vi "Re-Populate Tree.vi"(8 "error in":errorcluster, 9 "Tags map":refnum<vi>, 10 "Data in":string[][](array[string]), 11 "TreeControl in":refnum<vi>) -> (0 "error out":errorcluster)   [LabVIEW 2025, in "CAN-LIN Raw Bus Capture UI.lvlib"]
uses:
  CAN-LIN Raw Bus Capture UI.lvlib
  <vilib>/Utility/error.llb/whitespace.ctl
  <vilib>/Utility/error.llb/Trim Whitespace One-Sided.vi
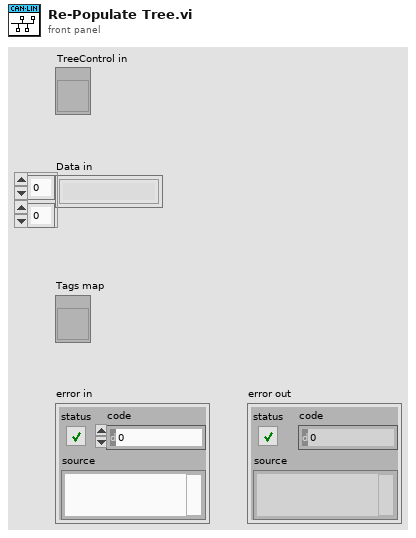
[diagram p1: front panel]
types:
  T1 = typedef "whitespace.ctl" = u16
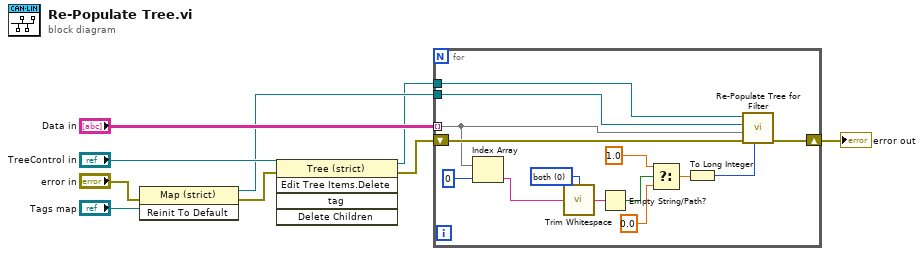
[diagram p0: block diagram]
diagram:
  n1 = invoke class="Map (strict)" method="Reinit To Default"(reference="Tags map", error in="error in") -> (reference out=w4:refnum<vi>, error out=w5:errorcluster)  [unwired: 1 in, 1 out]
  n2 = invoke class="Tree (strict)" method="Edit Tree Items.Delete"(reference="TreeControl in", error in=w5) -> (reference out=w3:refnum<vi>, error out=w2:errorcluster)  [unwired: 3 in, 3 out]
  n3 = for {
    tunnel: "Data in" -> [w13] mode=indexing
    tunnel: w4 -> [w11]
    tunnel: w3 -> [w12]
    shift-right: [w14] -> w1
    shift-left: w2 -> [w15]
    w20 = T1 0 items=["both", "start of string", "end of string"] ("location (both)")
    n4 = Index Array(array=w13, index=0) -> (element=w21:string)
    n5 = call <vilib>:"Trim Whitespace.vi"("string"=w21, "location (both)"=w20) -> ("trimmed string"=w22:string)
    n6 = Empty String/Path?(string/path=w22) -> (empty?=w19:bool)
    n7 = Select(t=1.0, s=w19, f=0.0) -> (s? t:f=w18:dbl)
    n8 = To Long Integer(number=w18) -> (32bit integer=w10:i32)
    n9 = call "Re-Populate Tree for Filter.vi"("Indent level"=w10, "error in"=w15, "Data in"=w13, "Tags map"=w11, "TreeControl in"=w12) -> ("error out"=w14:errorcluster)  [unwired: 6 in]
  }
  "error out" <- w1
